vi "Unregister Window.vi"(8 "error in (no error)":errorcluster caption="错误输入（无错误）", 10 "Window Name":string, 11 "User Interface 输入":refnum<class "User Interface.lvclass">) -> (0 "error out":errorcluster caption="错误输出", 3 "User Interface 输出":refnum<class "User Interface.lvclass">)   [LabVIEW 2018, in "MainInterface.lvlib" / "User Interface.lvclass"]
uses:
  User Interface.lvclass
  User Interface.lvclass/User Interface.ctl
  <vilib>/Delacor/Delacor QMH/Libraries/Message Queue_class/Delacor_lib_QMH_Message Queue.lvclass
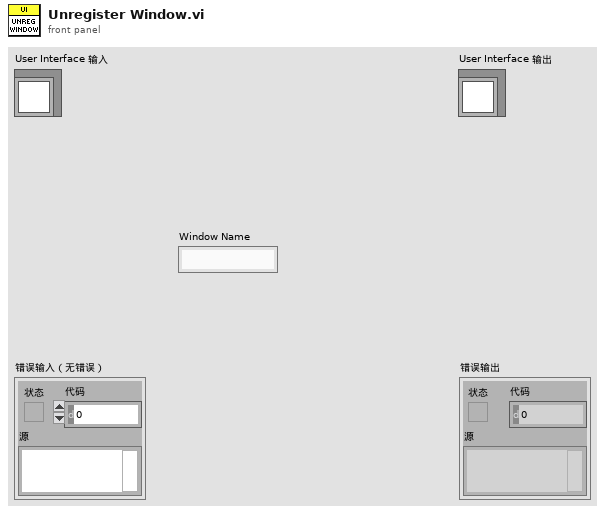
[diagram p1: front panel]
types:
  T1 = typedef "MainInterface.lvlib/Register Window Argument--cluster.ctl" = cluster{"Name":string, "Reference":refnum<vi>, "Message Queue":refnum<class "Delacor_lib_QMH_Message Queue.lvclass">}
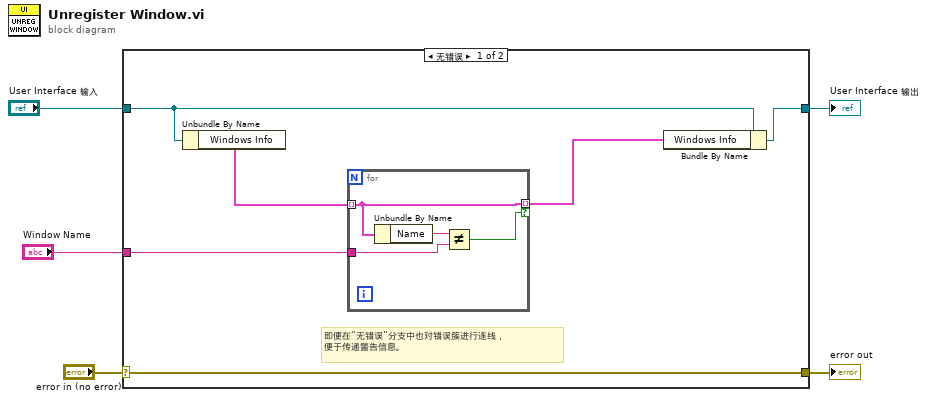
[diagram p0: block diagram]
diagram:
  n1 = case shown="无错误" "error in (no error)" {
    selector: "error in (no error)" -> [w11 w17]
    tunnel: [w11 w17] -> w4
    tunnel: [w8 w16] -> w2
    tunnel: "User Interface 输入" -> [w7 w16]
    tunnel: "Window Name" -> [w6 _]
    frame No Error {
      # "即便在“无错误”分支中也对错误簇进行连线，\n便于传递警告信息。"
      n2 = Unbundle By Name(w7) -> ("Windows Info"=w10:T1[])
      n3 = for {
        tunnel: w10 -> [w12] mode=indexing
        tunnel: w6 -> [w15]
        tunnel: [w12] -> w9 mode=indexing if=w14
        n4 = Unbundle By Name(w12) -> ("Name"=w13:string)
        n5 = Not Equal?(x=w13, y=w15) -> (x != y?=w14:bool)
      }
      n6 = Bundle By Name(cluster=w7, "Windows Info"=w9) -> (w8:refnum<class "User Interface.lvclass">)
    }
    frame Error {
    }
  }
  "error out" <- w4
  "User Interface 输出" <- w2
